vi "Read Protocol.vi"(8 "error in (no error)":errorcluster, 11 "navX - SERIAL in":refnum<class "navX - SERIAL.lvclass">) -> (0 "error out":errorcluster, 2 "Protocol":T1, 3 "navX - SERIAL out":refnum<class "navX - SERIAL.lvclass">)   [LabVIEW 2015, in "navX Library v3.lvlib" / "navX - SERIAL.lvclass"]
uses:
  navX - SERIAL.lvclass
  Protocol.ctl
  navX - SERIAL.lvclass/navX - SERIAL.ctl
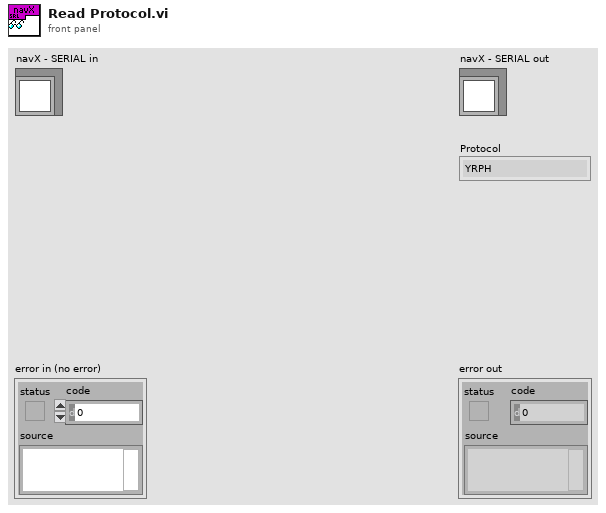
[diagram p1: front panel]
types:
  T1 = typedef "navX Library v3.lvlib/navX - SERIAL.lvclass/Protocol.ctl" = enum16{"YRPH", "Quaterinons", "Gyro/Raw", "AHRS", "AHRSAndPositioning"}
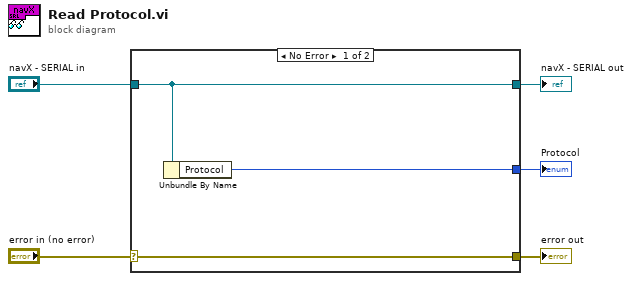
[diagram p0: block diagram]
diagram:
  n1 = case shown="No Error" "error in (no error)" {
    selector: "error in (no error)" -> [w8 w9]
    tunnel: [w8 w9] -> w4
    tunnel: [w7 w10] -> w2
    tunnel: "navX - SERIAL in" -> [w7 w10]
    tunnel: [w6 _] -> w1
    frame No Error {
      n2 = Unbundle By Name(w7) -> ("Protocol"=w6:T1)
    }
    frame Error {
    }
  }
  "error out" <- w4
  "navX - SERIAL out" <- w2
  "Protocol" <- w1
